vi "getSampleInfo.vi"(8 "error in (no error)":errorcluster, 11 "DeviceData in":refnum<class "DeviceData.lvclass">) -> (0 "error out":errorcluster, 1 "sampleRate":dbl, 2 "sampleNumber":i32, 3 "DeviceData out":refnum<class "DeviceData.lvclass">)   [LabVIEW 2011, in "DataMappers.lvlib" / "DeviceData.lvclass"]
uses:
  DeviceData.lvclass
  DeviceData.lvclass/DeviceData.ctl
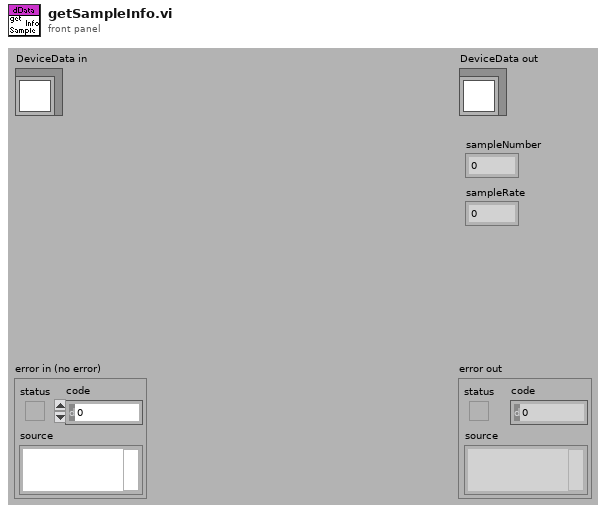
[diagram p1: front panel]
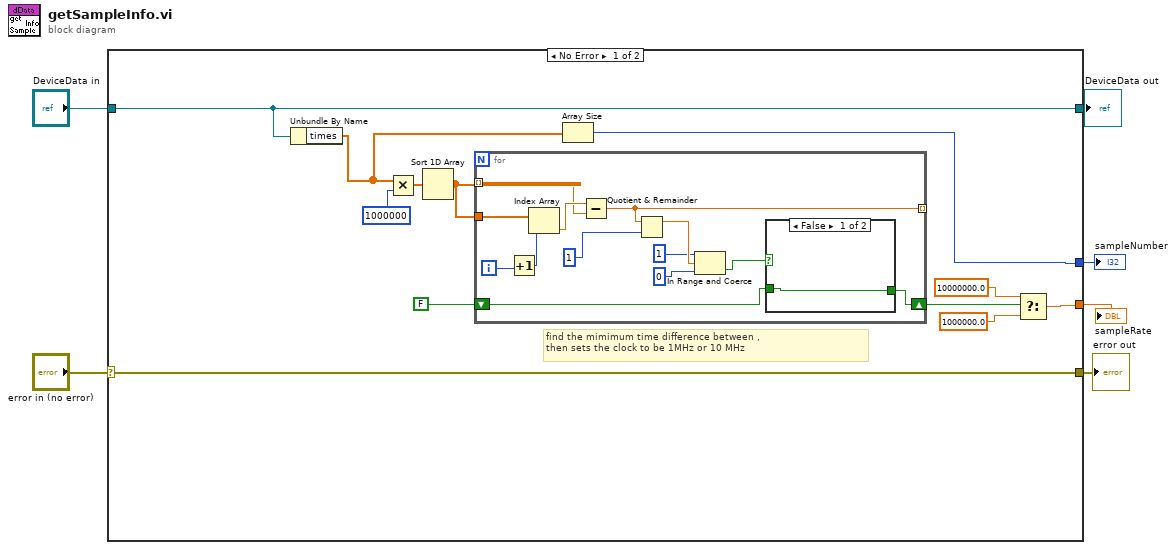
[diagram p0: block diagram]
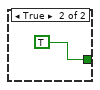
[diagram p2: hidden frame]
diagram:
  n1 = case shown="No Error" "error in (no error)" {
    selector: "error in (no error)" -> [w16 w35]
    tunnel: [w16 w35] -> w5
    tunnel: [w15 w34] -> w3
    tunnel: "DeviceData in" -> [w15 w34]
    tunnel: [w18 _] -> w2
    tunnel: [w17 _] -> w1
    frame No Error {
      # "find the mimimum time difference between ,\nthen sets the clock to be 1MHz or 10 MHz"
      n2 = Unbundle By Name(w15) -> ("times"=w7:dbl[])
      n3 = Multiply(x=w7, y=1000000) -> (x*y=w9:dbl[])
      n4 = Sort 1D Array(array=w9) -> (sorted array=w14:dbl[])
      n5 = for {
        tunnel: w14 -> [w27] mode=indexing
        tunnel: w14 -> [w31]
        tunnel: [w22] -> _ mode=indexing
        shift-right: [w19] -> w12
        shift-left: FALSE -> [w20]
        i -> [w30]
        n6 = Increment(x=w30) -> (x+1=w29:i32)
        n7 = Index Array(array=w31, index=w29) -> (element=w28:dbl)
        n8 = Subtract(x=w28, y=w27) -> (x-y=w22:dbl)
        n9 = Quotient & Remainder(x=w22, y=1) -> (x-y*floor(x/y)=w25:dbl)  [unwired: 1 out]
        n10 = In Range and Coerce(upper limit=1, x=w25, lower limit=0) -> (In Range?=w21:bool)  [unwired: 1 out]
        n11 = case shown="False" w21 {
          tunnel: w20 -> [w32 _]
          tunnel: [w32 TRUE] -> w19
          frame False {
          }
          frame True {
          }
        }
      }
      n12 = Array Size(array=w7) -> (size(s)=w18:i32)
      n13 = Select(t=10000000.0, s=w12, f=1000000.0) -> (s? t:f=w17:dbl)
    }
    frame Error {
    }
  }
  "error out" <- w5
  "DeviceData out" <- w3
  "sampleNumber" <- w2
  "sampleRate" <- w1
